vi "Get All Properties.vi"(0 "video in":refnum<class "MSC Video.lvclass">, 1 "precision":i16, 5 "error in (no error)":errorcluster) -> (14 "video out":refnum<class "MSC Video.lvclass">, 15 "Properties":string[][](array[string]), 19 "error out":errorcluster)   [LabVIEW 2014, in "MSC Video.lvclass"]
doc: "Returns all available properties as 2d string array."
uses:
  MSC Video.lvclass
  controls/Stream Property.ctl
  <userlib>/_OpenG.lib/array/array.llb/Delete Elements from 1D Array (Variant)__ogtk.vi
panel:
  in  "Dummy Camera Stream Property":T1=3 caption="Camera Stream Property" items=["Position msec", "Position frames", "Position avi ratio", "Frame Width", "Frame Height", "FPS", "FourCC codec", "Frame Count", "Format", "Mode", "Brightness", "Contrast", "Saturation", "Hue", "Gain", "Exposure", "Convert RGB", "White Balance U", "Rectification", "Monochrome", "Sharpness", "Auto Exposure", "Gamma", "Temperature", "Trigger", "Trigger Delay", "White Balance V", "Zoom", "Focus", "Guid", "ISO Speed", "Max DV1394", "Backlight", "Pan", "Tilt", "Rolls", "Iris", "Settings", "Buffersize"]
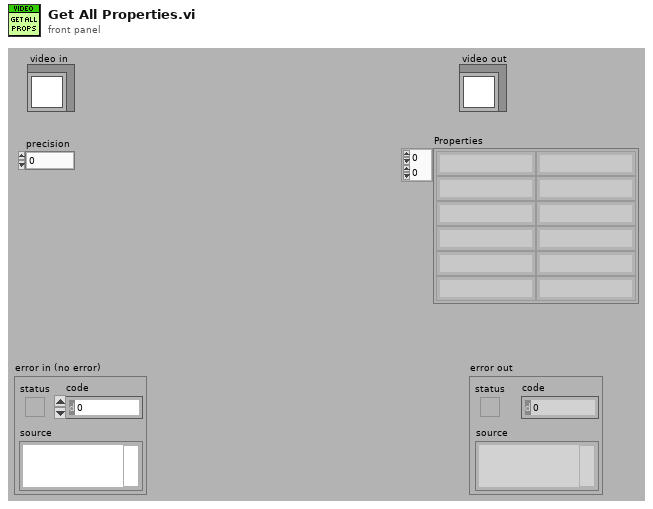
[diagram p1: front panel]
types:
  T1 = typedef "MSC Video.lvclass/Stream Property.ctl" = u16
  T2 = typedef "LVStringsAndValuesArrayTypeDef_U16.ctl" = cluster{"String":string, "Value":u16}[]
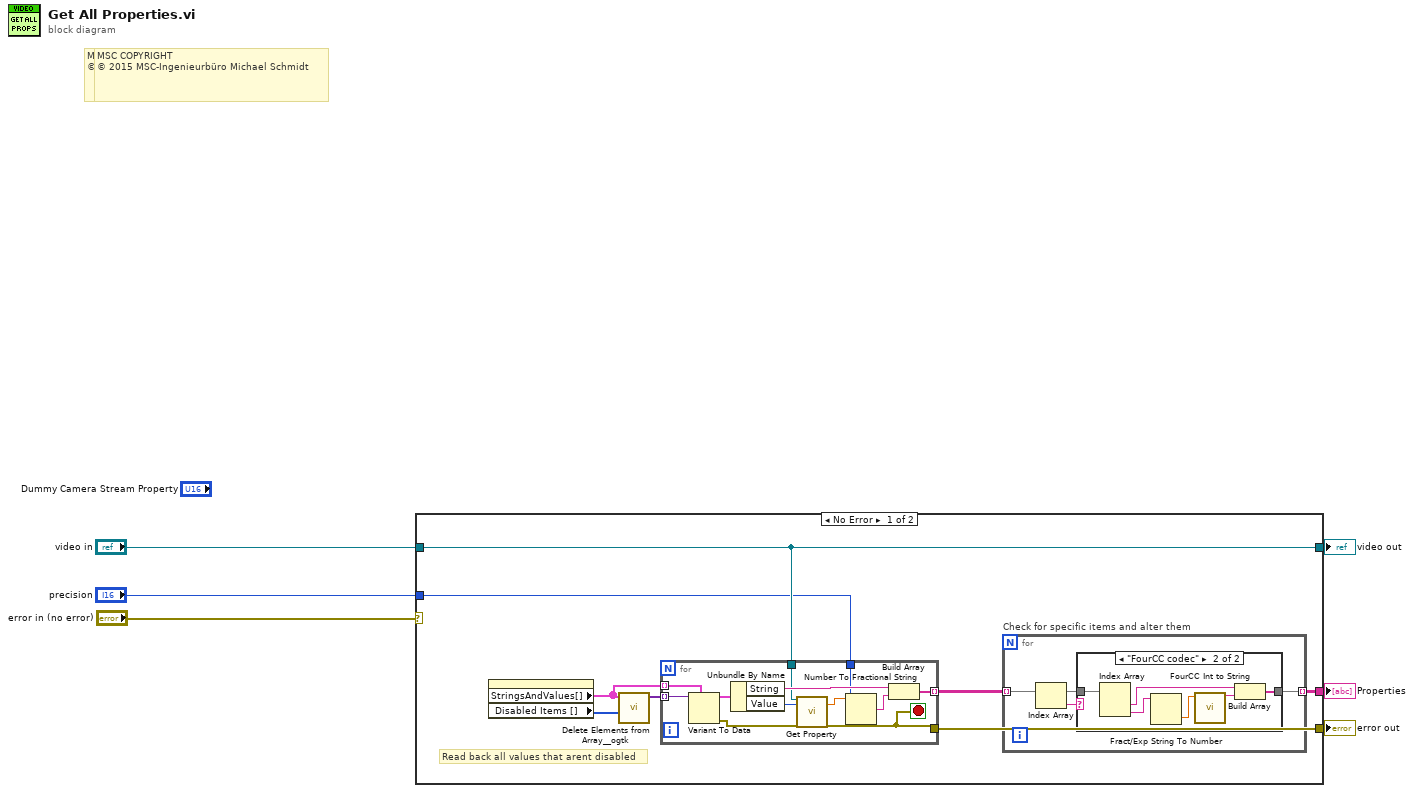
[diagram p0: block diagram]
diagram:
  # "MSC COPYRIGHT\n© 2016 MSC-Ingenieurbüro Michael Schmidt"
  # "MSC COPYRIGHT\n© 2016 MSC-Ingenieurbüro Michael Schmidt"
  # "MSC COPYRIGHT\n© 2015 MSC-Ingenieurbüro Michael Schmidt"
  n1 = case shown="No Error" "error in (no error)" {
    selector: "error in (no error)" -> [_ w38]
    tunnel: [w9 w38] -> w5
    tunnel: [w11 w37] -> w3
    tunnel: "video in" -> [w11 w37]
    tunnel: "precision" -> [w10 _]
    tunnel: [w7 _] -> w1
    frame No Error {
      # "Read back all values that arent disabled"
      n2 = property on="Dummy Camera Stream Property" class="Ring (strict)"() -> ("StringsAndValues[]"=w14:T2, "Disabled Items []"=w12:i32[])  [unwired: 2 in, 2 out]
      n3 = call-poly <userlib>:"Delete Elements from Array__ogtk.vi"("indices"=w12, "array"=w14) -> ("array w/ subset deleted"=w13:variant[])  [unwired: 8 in, 1 out]
      n4 = for {
        tunnel: w13 -> [w36] mode=indexing
        tunnel: w14 -> [w35] mode=indexing
        tunnel: w11 -> [w31]
        tunnel: w10 -> [w29]
        tunnel: [w27] -> w8 mode=indexing
        tunnel: [w26] -> w9
        stop <- w26 stop-if-true
        n5 = Variant To Data(type=w35, Variant=w36) -> (data=w34:cluster{"String":string, "Value":u16}, error out=w25:errorcluster)  [unwired: 1 in]
        n6 = Unbundle By Name(w34) -> ("String"=w33:string, "Value"=w32:u16)
        n7 = call-dynamic "Get Property.vi"("video in"=w31, "Camera Stream Property"=w32, "error in (no error)"=w25) -> ("propertyValue"=w30:dbl, "error out"=w26:errorcluster)  [unwired: 14 in, 1 out]
        n8 = Number To Fractional String(number=w30, precision (6)=w29) -> (F-format string=w28:string)  [unwired: 2 in]
        n9 = Build Array(w33, w28) -> (w27:string[])
      }
      n10 = for "Check for specific items and alter them" {
        tunnel: w8 -> [w16] mode=indexing
        tunnel: [w15] -> w7 mode=indexing
        n11 = Index Array(array=w16) -> (element=w17:string)  [unwired: 1 in]
        n12 = case shown="\"FourCC codec\"" w17 {
          tunnel: w16 -> [w18 w24]
          tunnel: [w18 w21] -> w15
          frame Default {
          }
          frame "FourCC codec" {
            n13 = Index Array(array=w24) -> (element #1=w22:string, element #2=w20:string)  [unwired: 2 in]
            n14 = Fract/Exp String To Number(string=w20) -> (number=w19:dbl)  [unwired: 3 in, 1 out]
            n15 = call "FourCC Int to String.vi"("fourCC Int"=w19) -> ("fourCC String"=w23:string)  [unwired: 9 in, 1 out]
            n16 = Build Array(w22, w23) -> (w21:string[])
          }
        }
      }
    }
    frame Error {
    }
  }
  "error out" <- w5
  "video out" <- w3
  "Properties" <- w1
